vi "process safe state.vi"(8 "error in":errorcluster, 9 "result allocation":T1, 10 "parameters":T1, 11 "Simple Sequencer TBM runtime in":refnum<class "Simple Sequencer TBM runtime.lvclass">) -> (0 "error out":errorcluster, 1 "results":T1, 2 "parameter allocation":T1, 3 "Simple Sequencer TBM runtime out":refnum<class "Simple Sequencer TBM runtime.lvclass">)   [LabVIEW 2014, in "Simple Sequencer TBM runtime.lvclass"]
doc: "Provides an interface for information processing by a module when in a safe state. This interface simply calls the normal processing function. However, if child modules need to have custom logic during safe-state operation, this can be implemented here.\nNI Tag Bus Module Framework 1.0.2.34\nNI Systems Engineering"
uses:
  Simple Sequencer TBM runtime.lvclass
  <vilib>/NI/Tag Bus/table/data table.ctl
  Simple Sequencer TBM runtime.lvclass/Simple Sequencer TBM runtime.ctl
  <vilib>/NI/Tag Bus/table/data table.lvlib
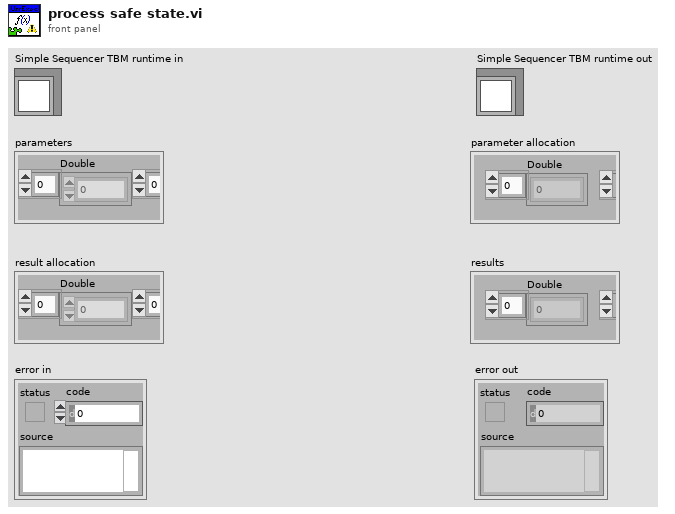
[diagram p1: front panel]
types:
  T1 = typedef "tag bus.lvlib/data table.lvlib/data table.ctl" = cluster{"Double":dbl[], "Single":sgl[], "I64":i64[], "I32":i32[], "I16":i16[], "I8":i8[], "U64":u64[], "U32":u32[], "U16":u16[], "U8":u8[], "Boolean":bool[], "String":string[], "Array of Double":cluster{"DBL Array":dbl[]}[], "Array of Single":cluster{"SGL Array":sgl[]}[], "Array of I64":cluster{"I64 Array":i64[]}[], "Array of I32":cluster{"I32 Array":i32[]}[], "Array of I16":cluster{"I16 Array":i16[]}[], "Array of I8":cluster{"I8 Array":i8[]}[], "Array of U64":cluster{"U64 Array":u64[]}[], "Array of U32":cluster{"U32 Array":u32[]}[], "Array of U16":cluster{"U16 Array":u16[]}[], "Array of U8":cluster{"U8 Array":u8[]}[], "Array of Boolean":cluster{"Boolean Array":bool[]}[], "Array of String":cluster{"String Array":string[]}[]}
  T2 = typedef "Simple Sequencer TBM runtime.lvclass/actions with configuration.ctl" = cluster{"action":refnum<class "action.lvclass">, "parameters":T1, "parameters specification":T3[], "results":T1, "results specification":T3[]}
  T3 = typedef "tag bus.lvlib/data table.lvlib/transfer specification.ctl" = cluster{"data type":T4, "sink indices":i32[], "source indices":i32[]}
  T4 = typedef "tag bus.lvlib/tag descriptor.lvclass/Data Type.ctl" = enum16{"Double", "Single", "I64", "I32", "I16", "I8", "U64", "U32", "U16", "U8", "Boolean", "String", "Array of Double", "Array of Single", "Array of I64", "Array of I32", "Array of I16", "Array of I8", "Array of U64", "Array of U32", "Array of U16", "Array of U8", "Array of Boolean", "Array of String"}
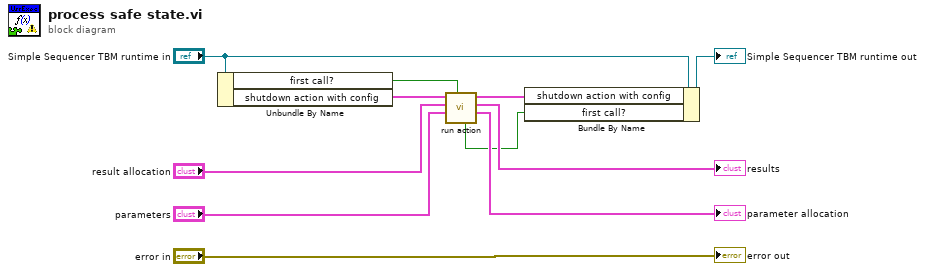
[diagram p0: block diagram]
diagram:
  n1 = Unbundle By Name("Simple Sequencer TBM runtime in") -> ("first call?"=w7:bool, "shutdown action with config"=w6:T2)
  n2 = call "run action.vi"("first call?"=w7, "result allocation"="parameters", "parameters"="result allocation", "action with configuration"=w6) -> ("results"=→"parameter allocation":T1, "parameters allocation"=→"results":T1, "action with configuration out"=w4:T2, "complete?"=w3:bool)  [unwired: 3 in, 1 out]
  n3 = Bundle By Name(cluster="Simple Sequencer TBM runtime in", "shutdown action with config"=w4, "first call?"=w3) -> (→"Simple Sequencer TBM runtime out":refnum<class "Simple Sequencer TBM runtime.lvclass">)
  "error out" <- "error in"
